vi "Change Variant by Menu Tag.vi"(8 "error in (no error)":errorcluster, 10 "tag":string, 11 "Cluster":variant) -> (0 "error out":errorcluster, 1 "Cluster Changed":bool, 2 "Item":string, 3 "VCluster out":variant)   [LabVIEW 2020, in "Menu From Cluster.lvlib"]
doc: "Takes a tag (set previously be \"Add Item to Menu\") and sets the corresponding item in the supplied variant. Allowed types are enums, booleans, or clusters of such types."
uses:
  <vilib>/JDP Science/JDP Science Common Utilities/Shortcut Menu Tools/Menu From Cluster.lvlib
  <vilib>/Utility/VariantDataType/VariantType.lvlib
  <vilib>/JDP Science/JDP Science Common Utilities/JDP Utility.lvlib
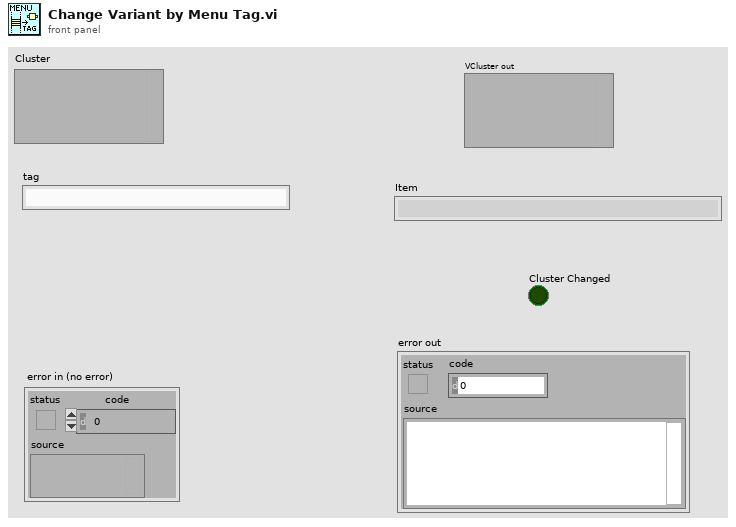
[diagram p1: front panel]
types:
  T1 = typedef "VariantType.lvlib/Type.ctl" = enum8{"Invalid Type", "Void", "I8", "I16", "I32", "I64", "U8", "U16", "U32", "U64", "Single Float", "Double Float", "Extended Float", "Single Complex", "Double Complex", "Extended Complex", "Enum U8", "Enum U16", "Enum U32", "Enum U64", "Single Float With Unit", "Double Float With Unit", "Extended Float With Unit", "Single Complex with Unit", "Double Complex with Unit", "Extended Complex with Unit", "Boolean", "String", "Path", "Picture", "Tag", "Array", "Cluster", "Variant", "LV Variant", "Waveform", "Timestamp", "Digital Waveform", "Digital Data", "ExpressData", "Refnum", "External Data", "VI", "Poly VI", "LabVIEW Class Instance", "Fixed Point"}
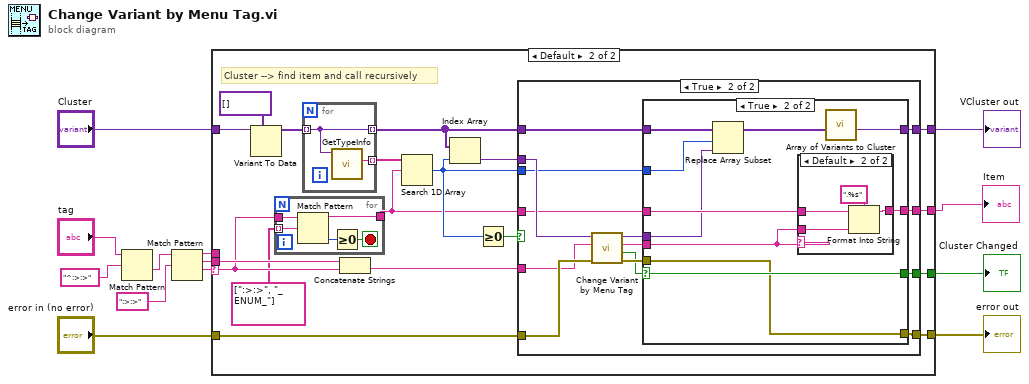
[diagram p0: block diagram]
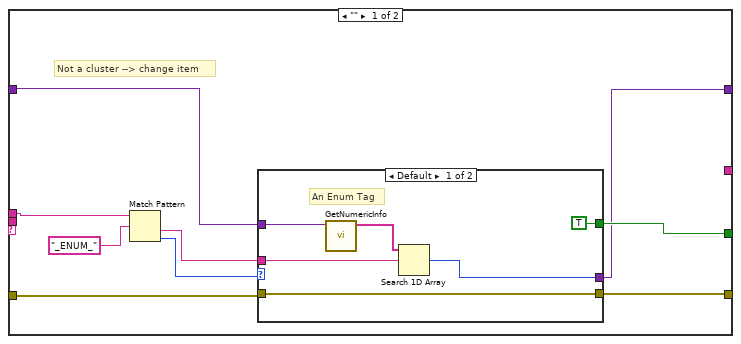
[diagram p2: hidden frame]
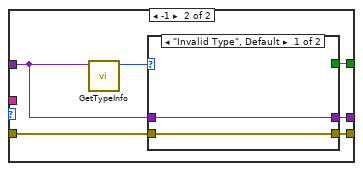
[diagram p3: hidden frame]
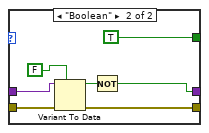
[diagram p4: hidden frame]
diagram:
  n1 = Match Pattern(string="tag", regular expression="^:>:>") -> (after substring=w7:string)  [unwired: 4 out]
  n2 = Match Pattern(string=w7, regular expression=":>:>") -> (before substring=w4:string, match substring=w3:string, after substring=w6:string)  [unwired: 2 out]
  n3 = case shown="Default" w6 {
    selector: w6 -> [_ w46]
    tunnel: [w15 w56] -> w13
    tunnel: [w17 w61] -> w12
    tunnel: "Cluster" -> [w14 w53]
    tunnel: [w16 w60] -> w10
    tunnel: "error in (no error)" -> [w19 w55]
    tunnel: w4 -> [w18 _]
    tunnel: w3 -> [_ w58]
    tunnel: [_ w57] -> w2
    frame "" {
      # "Not a cluster --> change item"
      n4 = Match Pattern(string=w18, regular expression="_ENUM_" ("format string")) -> (after substring=w20:string, offset past match=w21:i32)  [unwired: 3 out]
      n5 = case shown="Default" w21 {
        tunnel: w20 -> [w24 _]
        tunnel: w14 -> [w26 w29]
        tunnel: [w23 w34] -> w15
        tunnel: [w28 w33] -> w17
        tunnel: [TRUE w31] -> w16
        tunnel: w19 -> [w28 w32]
        frame Default {
          # "An Enum Tag"
          n6 = call <vilib>:"GetNumericInfo.vi"("Variant"=w26) -> ("EnumNames"=w25:string[])  [unwired: 7 in, 3 out]
          n7 = Search 1D Array(1D array=w25, element=w24) -> (index of element=w23:i32)  [unwired: 1 in]
        }
        frame -1 {
          n8 = call <vilib>:"GetTypeInfo.vi"("Variant"=w29) -> ("Type Enum"=w30:T1)  [unwired: 6 in, 4 out]
          n9 = case shown="\"Invalid Type\", Default" w30 {
            tunnel: w29 -> [w35 w42]
            tunnel: [w35 w38] -> w34
            tunnel: [w36 w37] -> w33
            tunnel: w32 -> [w36 w40]
            tunnel: [_ TRUE] -> w31
            frame "Invalid Type", Default {
            }
            frame "Boolean" {
              n10 = Variant To Data(error in=w40, type=FALSE, Variant=w42) -> (data=w41:bool, error out=w37:errorcluster)
              n11 = Not(x=w41) -> (.not. x?=w38:bool)
            }
          }
        }
      }
    }
    frame Default {
      # "Cluster --> find item and call recursively"
      n12 = Variant To Data(type=variant[] [], Variant=w53) -> (data=w52:variant[])  [unwired: 1 in, 1 out]
      n13 = for {
        tunnel: w46 -> [w66]
        tunnel: [w65] -> w45
        tunnel: string[] [":>:>", "_ENUM_"] -> [w64] mode=indexing
        stop <- w63 stop-if-true
        n14 = Match Pattern(string=w66, regular expression=w64) -> (before substring=w65:string, offset past match=w62:i32)  [unwired: 1 in, 2 out]
        n15 = Greater Or Equal To 0?(x=w62) -> (x >= 0?=w63:bool)
      }
      n16 = for {
        tunnel: [w68] -> w50 mode=indexing
        tunnel: w52 -> [w68] mode=indexing
        tunnel: [w67] -> w51 mode=indexing
        n17 = call <vilib>:"GetTypeInfo.vi"("Variant"=w68) -> ("Name"=w67:string)  [unwired: 6 in, 4 out]
      }
      n18 = Concatenate Strings(w58, w46) -> (w59:string)
      n19 = Search 1D Array(1D array=w51, element=w45) -> (index of element=w47:i32)  [unwired: 1 in]
      n20 = Index Array(array=w50, index=w47) -> (element=w49:variant)
      n21 = Greater Or Equal To 0?(x=w47) -> (x >= 0?=w48:bool)
      n22 = case shown="True" w48 {
        tunnel: [w69 w84] -> w61
        tunnel: w50 -> [w70 w83]
        tunnel: [_ w72] -> w60
        tunnel: w49 -> [_ w82]
        tunnel: w55 -> [w69 w81]
        tunnel: w59 -> [_ w78]
        tunnel: [_ w77] -> w57
        tunnel: [w70 w76] -> w56
        tunnel: w45 -> [_ w75]
        tunnel: w47 -> [_ w71]
        frame False {
        }
        frame True {
          n23 = call <vilib>:"Change Variant by Menu Tag.vi"("error in (no error)"=w81, "tag"=w78, "Cluster"=w82) -> ("error out"=w79:errorcluster, "Cluster Changed"=w73:bool, "Item"=w74:string, "VCluster out"=w80:variant)  [unwired: 5 in]
          n24 = case shown="True" w73 {
            selector: w73 -> [w86 w94]
            tunnel: [w85 w88] -> w84
            tunnel: w83 -> [w87 w93]
            tunnel: w80 -> [_ w91]
            tunnel: w79 -> [w85 w88]
            tunnel: [_ w97] -> w77
            tunnel: [w87 w89] -> w76
            tunnel: w75 -> [_ w96]
            tunnel: w74 -> [_ w95]
            tunnel: [w86 w94] -> w72
            tunnel: w71 -> [_ w92]
            frame False {
            }
            frame True {
              n25 = Replace Array Subset(array=w93, new element=w91, index=w92) -> (w90:variant[])
              n26 = case shown="Default" w95 {
                tunnel: [w98 w102] -> w97
                tunnel: w95 -> [_ w100]
                tunnel: w96 -> [w98 w99]
                frame "" {
                }
                frame Default {
                  n27 = Format Into String(format string=".%s", initial string=w99, w100) -> (resulting string=w102:string)  [unwired: 1 in, 1 out]
                }
              }
              n28 = call <vilib>:"Array of Variants to Cluster.vi"("Array of Variants"=w90) -> ("Cluster of Variants"=w89:variant)  [unwired: 10 in]
            }
          }
        }
      }
    }
  }
  "VCluster out" <- w13
  "error out" <- w12
  "Cluster Changed" <- w10
  "Item" <- w2
